vi "Edit Config.vi"(8 "error in (no error)":errorcluster, 11 "Lookup Table in":refnum<class "Lookup Table.lvclass">) -> (0 "error out":errorcluster, 3 "Lookup Table out":refnum<class "Lookup Table.lvclass">)   [LabVIEW 2018, in "Lookup Table.lvclass"]
doc: "Lookup Table.lvclass:Edit Config.vi\n\nThis VI is the configuration editor user interface for the Lookup Table class.\n\nInstrument Communication Module Version 1.0\nSeptember, 2017 Original Code Consulting David Thomson\n www.originalcode.com"
uses:
  Lookup Table.lvclass
  ICM Editor Command.ctl
  ICM Class Editor State.ctl
  ICM Config Command.ctl
  Lookup Table.lvclass/Lookup Table.ctl
panel:
  in  "Export":bool
  in  "Import":bool
  in  "New Instance":string
  in  "Delete":bool
  in  "Add":bool
  in  "Revert Scaling":bool
  in  "Table":cluster{"Raw Value":dbl, "Scaled Value":dbl}[](array[cluster])
  in  "Instance":u16(ring) items=["table", "hello"]
  in  "Save":bool
  # "To Add New Scaling Instance:\n1. Enter name in New Instance control to the right\n2. Click Add New Button\n3. Select Name in Instance control to the left\n4. Edit table below"
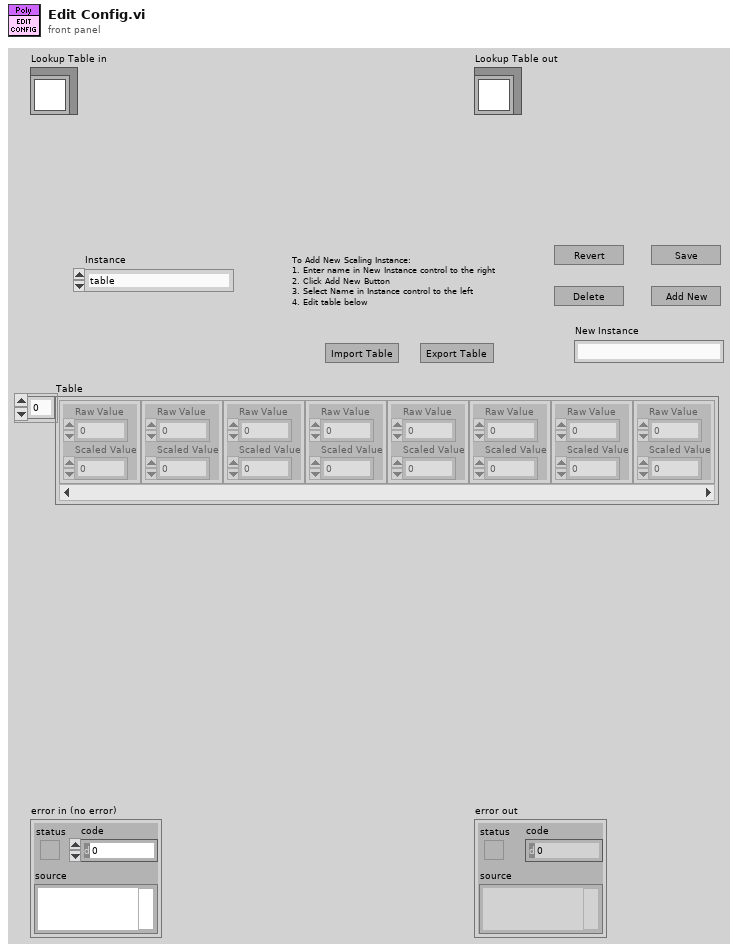
[diagram p1: front panel]
types:
  T1 = typedef "ICM Config Command.ctl" = enum16{"No-op", "Re-Display Sc."}
  T2 = typedef "ICM Class Editor State.ctl" = enum16{"Init", "Wait", "Write", "Read", "Display", "Set Flashing", "Error", "Stop"}
  T3 = typedef "ICM Editor Command.ctl" = enum16{"No-op", "Exit"}
  T4 = enum8{"Enabled", "Disabled", "Disabled and Grayed Out"}
  T5 = cluster{"Instance":string, "Table":cluster{"Raw Value":dbl, "Sca;ed Value":dbl}[]}
  T6 = cluster{"Instance":string, "Table":cluster{"Raw Value":dbl, "Scaled Value":dbl}[]}[]
  T7 = cluster{"RingText.Text":string, "Table":cluster{"Raw Value":dbl, "Scaled Value":dbl}[]}
  T8 = cluster{"Instance":string, "Table":cluster{"Raw Value":dbl, "Sca;ed Value":dbl}[]}[]
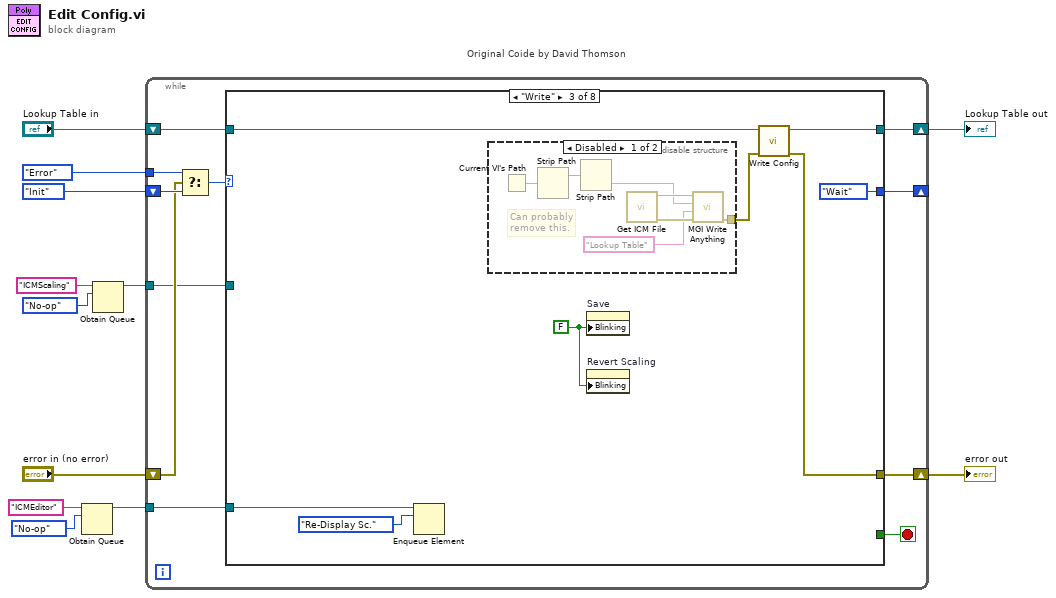
[diagram p0: block diagram]
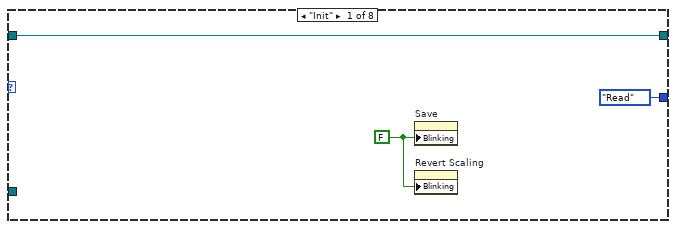
[diagram p2: hidden frame]
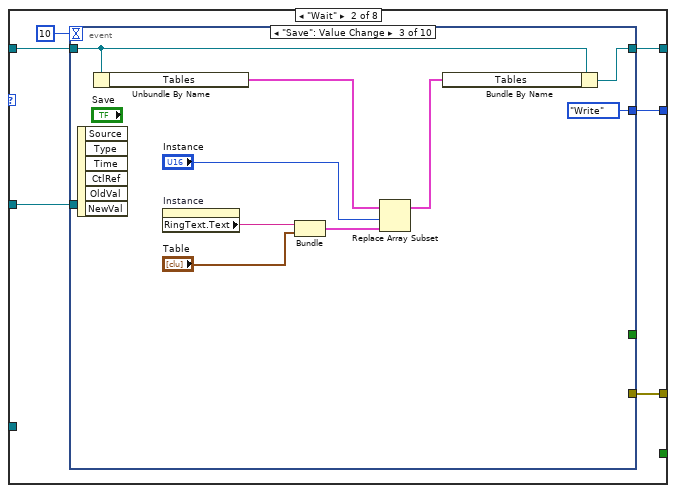
[diagram p3: hidden frame]
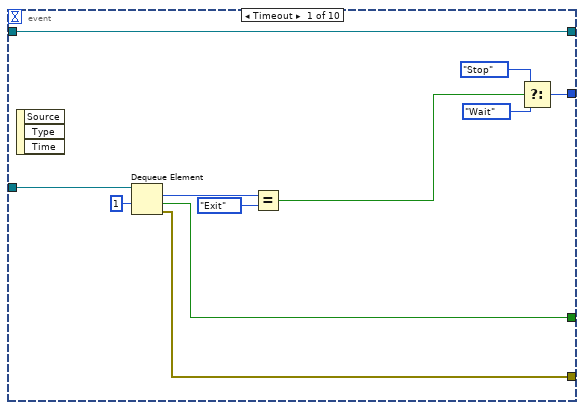
[diagram p4: hidden frame]
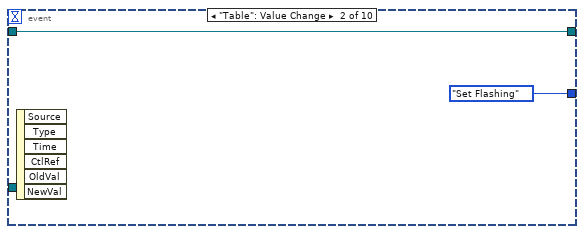
[diagram p5: hidden frame]
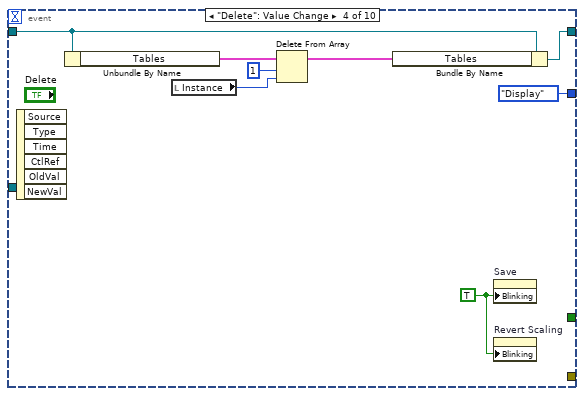
[diagram p6: hidden frame]
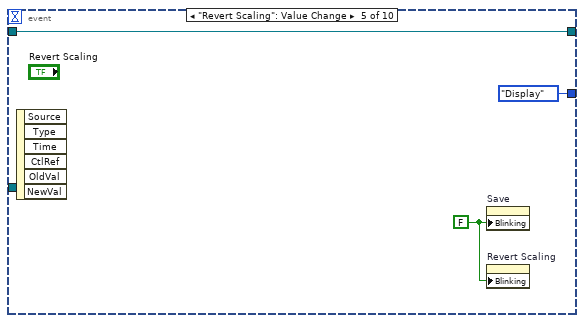
[diagram p7: hidden frame]
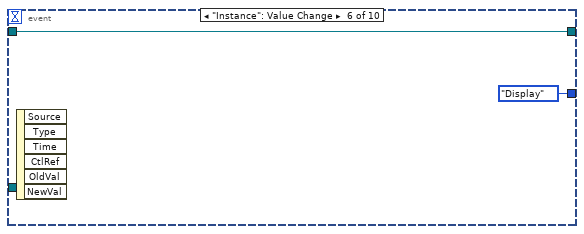
[diagram p8: hidden frame]
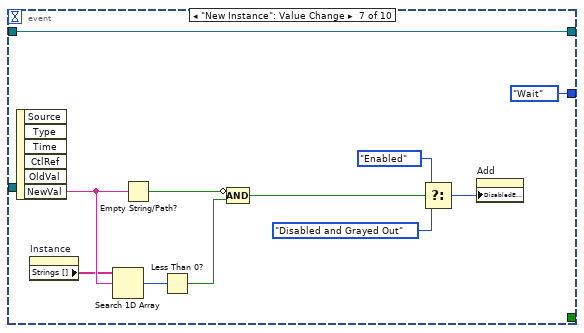
[diagram p9: hidden frame]
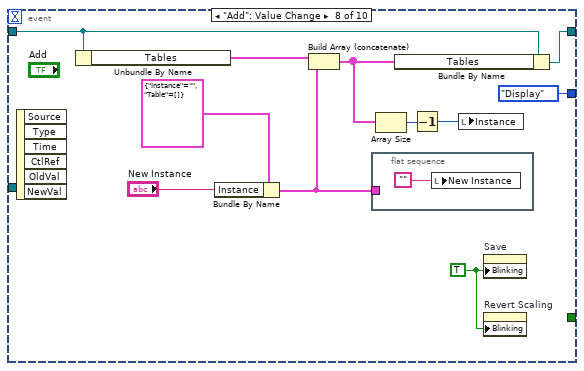
[diagram p10: hidden frame]
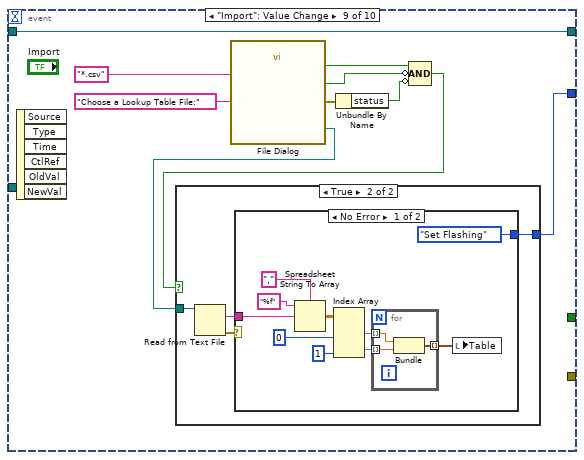
[diagram p11: hidden frame]
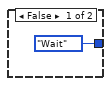
[diagram p12: hidden frame]
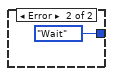
[diagram p13: hidden frame]
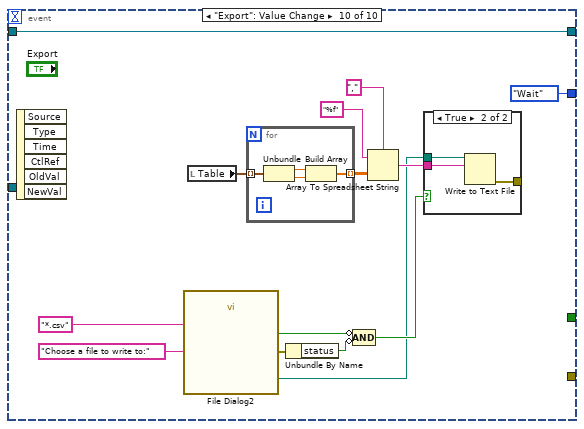
[diagram p14: hidden frame]
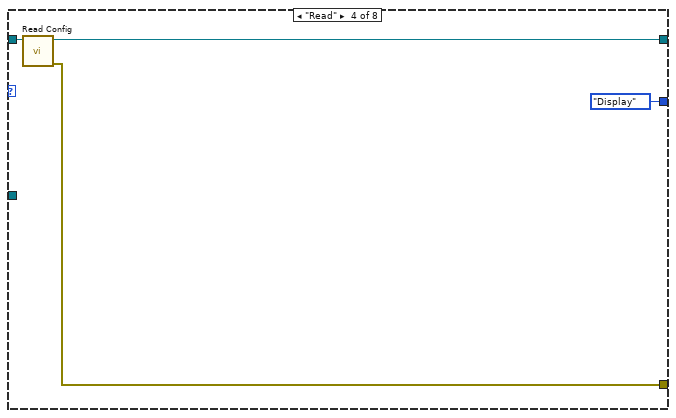
[diagram p17: hidden frame]
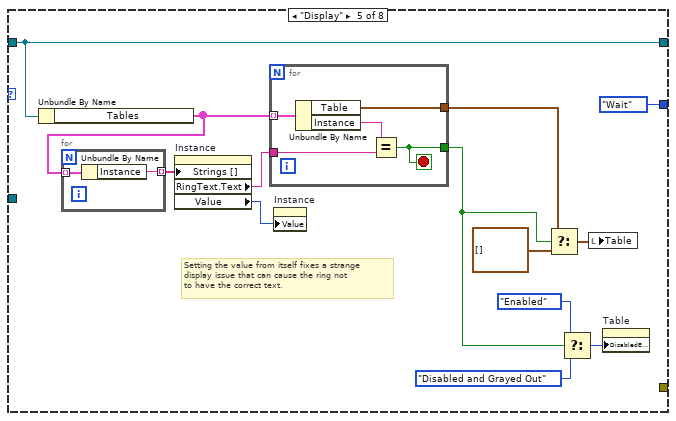
[diagram p18: hidden frame]
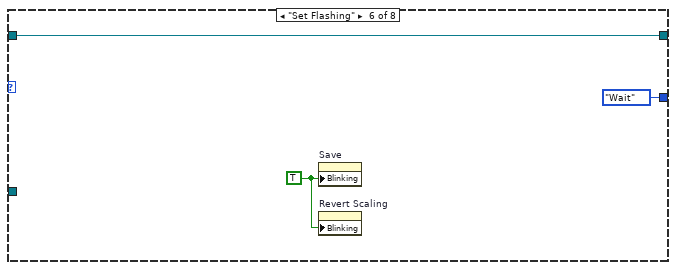
[diagram p19: hidden frame]
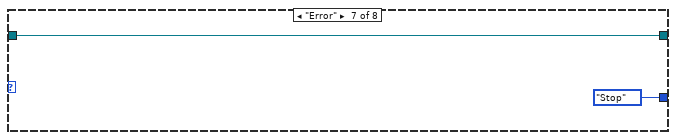
[diagram p20: hidden frame]
diagram:
  n1 = Obtain Queue(name (unnamed)="ICMEditor", element data type=ICM_Config_Command."No-op" ("Editor Command")) -> (queue out=w1:refnum<queue>)  [unwired: 3 in, 2 out]
  n2 = Obtain Queue(name (unnamed)="ICMScaling", element data type=ICM_Editor_Command."No-op" ("Editor Command")) -> (queue out=w8:refnum<queue>)  [unwired: 3 in, 2 out]
  n3 = while "Original Coide by David Thomson" {
    shift-right: [w23] -> w11
    shift-left: "Lookup Table in" -> [w22]
    shift-right: [w16] -> _
    shift-left: ICM_Class_Editor_State."Init" ("Config State") -> [w20]
    shift-right: [w15] -> w4
    shift-left: "error in (no error)" -> [w18]
    tunnel: ICM_Class_Editor_State."Error" ("Config State") -> [w17]
    tunnel: w8 -> [w14]
    tunnel: w1 -> [w13]
    stop <- w21 stop-if-true
    n4 = Select(t=w17, s=w18, f=w20) -> (s? t:f=w19:T2)
    n5 = case shown="\"Write\"" w19 {
      tunnel: [w25 w30 w147 w156 w168 w182 w184 w187] -> w23
      tunnel: w22 -> [w25 w29 w144 w158 w168 w182 w184 w187]
      tunnel: [_ _ _ _ _ _ _ TRUE] -> w21
      tunnel: [ICM_Class_Editor_State."Read" ("Config State") w31 ICM_Class_Editor_State."Wait" ("Config State") ICM_Class_Editor_State."Display" ("Config State") ICM_Class_Editor_State."Wait" ("Config State") ICM_Class_Editor_State."Wait" ("Config State") ICM_Class_Editor_State."Stop" ("Config State") ICM_Class_Editor_State."Stop" ("Config State")] -> w16
      tunnel: [_ w27 w146 w157 _ _ _ _] -> w15
      tunnel: w14 -> [_ w28 _ _ _ _ _ _]
      tunnel: w13 -> [_ _ w141 _ _ _ _ _]
      frame "Init" {
        w24 = FALSE ("Blinking")
        n6 = property on="Save" class="Bool"("Blinking"=w24) -> ()  [unwired: 2 in, 2 out]
        n7 = property on="Revert Scaling" class="Bool"("Blinking"=w24) -> ()  [unwired: 2 in, 2 out]
      }
      frame "Wait" {
        n8 = event shown="[2] \"Save\": Value Change" {
          selector: _ -> [_ _ _ _ _ _ _ _ _ _]
          dyn-events: _ -> [_ _ _ _ _ _ _ _ _ _]
          timeout: 10 -> [_ _ _ _ _ _ _ _ _ _]
          tunnel: [w40 ICM_Class_Editor_State."Set Flashing" ("Config State") ICM_Class_Editor_State."Write" ("Config State") ICM_Class_Editor_State."Display" ("Config State") ICM_Class_Editor_State."Display" ("Config State") ICM_Class_Editor_State."Display" ("Config State") ICM_Class_Editor_State."Wait" ("Config State") ICM_Class_Editor_State."Display" ("Config State") w91 ICM_Class_Editor_State."Wait" ("Config State")] -> w31
          tunnel: [w43 w45 w53 w57 w65 w67 w78 w87 w100 w133] -> w30
          tunnel: w29 -> [w43 w45 w52 w58 w65 w67 w78 w88 w100 w133]
          tunnel: w28 -> [w42 _ _ _ _ _ _ _ _ _]
          tunnel: [w34 _ _ _ _ _ _ _ _ _] -> w27
          tunnel: [w33 _ _ _ _ _ _ _ _ _] -> _
          event Timeout {
            n9 = event-data() -> ()  [unwired: 1 in, 3 out]
            n10 = Dequeue Element(queue=w42, timeout in ms (-1)=1) -> (element=w39:T3, timed out?=w33:bool, error out=w34:errorcluster)  [unwired: 1 in, 1 out]
            n11 = Equal?(x=w39, y=ICM_Editor_Command."Exit") -> (x = y?=w37:bool)
            n12 = Select(t=ICM_Class_Editor_State."Stop" ("Config State"), s=w37, f=ICM_Class_Editor_State."Wait" ("Config State")) -> (s? t:f=w40:T2)
          }
          event "Table": Value Change {
            n13 = event-data() -> ()  [unwired: 1 in, 6 out]
          }
          event "Save": Value Change {
            n14 = event-data() -> ()  [unwired: 1 in, 6 out]
            n15 = Unbundle By Name(w52) -> ("Tables"=w50:T6)
            n16 = property on="Instance" class="Ring (strict)"() -> ("RingText.Text"=w47:string)  [unwired: 2 in, 2 out]
            n17 = Bundle("RingText.Text"=w47, "Table"="Table") -> (w51:T7)  [unwired: 1 in]
            n18 = Replace Array Subset(array=w50, new element=w51, index="Instance") -> (w49:T6)
            n19 = Bundle By Name(cluster=w52, "Tables"=w49) -> (w53:refnum<class "Lookup Table.lvclass">)
          }
          event "Delete": Value Change {
            w62 = TRUE ("Blinking")
            n20 = event-data() -> ()  [unwired: 1 in, 6 out]
            n21 = Unbundle By Name(w58) -> ("Tables"=w59:T6)
            n22 = local read "Instance"() -> (w56:u16)
            n23 = Delete From Array(array=w59, length=1, index=w56) -> (array with subset deleted=w61:T6)  [unwired: 1 out]
            n24 = Bundle By Name(cluster=w58, "Tables"=w61) -> (w57:refnum<class "Lookup Table.lvclass">)
            n25 = property on="Save" class="Bool"("Blinking"=w62) -> ()  [unwired: 2 in, 2 out]
            n26 = property on="Revert Scaling" class="Bool"("Blinking"=w62) -> ()  [unwired: 2 in, 2 out]
          }
          event "Revert Scaling": Value Change {
            w63 = FALSE ("Blinking")
            n27 = event-data() -> ()  [unwired: 1 in, 6 out]
            n28 = property on="Save" class="Bool"("Blinking"=w63) -> ()  [unwired: 2 in, 2 out]
            n29 = property on="Revert Scaling" class="Bool"("Blinking"=w63) -> ()  [unwired: 2 in, 2 out]
          }
          event "Instance": Value Change {
            n30 = event-data() -> ()  [unwired: 1 in, 6 out]
          }
          event "New Instance": Value Change {
            n31 = event-data() -> ("NewVal"=w70:string)  [unwired: 1 in, 5 out]
            n32 = property on="Instance" class="Ring (strict)"() -> ("Strings []"=w68:string[])  [unwired: 2 in, 2 out]
            n33 = Search 1D Array(1D array=w68, element=w70) -> (index of element=w75:i32)  [unwired: 1 in]
            n34 = Empty String/Path?(string/path=w70) -> (empty?=w73:bool)
            n35 = Less Than 0?(x=w75) -> (x < 0?=w76:bool)
            n36 = Compound Arithmetic op=AND(invert w73, w76) -> (w74:bool)
            n37 = Select(t=T4."Enabled" ("Disabled"), s=w74, f=T4."Disabled and Grayed Out" ("Disabled")) -> (s? t:f=w69:T4)
            n38 = property on="Add" class="Bool"("DisabledEnum"=w69) -> ()  [unwired: 2 in, 2 out]
          }
          event "Add": Value Change {
            w83 = TRUE ("Blinking")
            n39 = event-data() -> ()  [unwired: 1 in, 6 out]
            n40 = Unbundle By Name(w88) -> ("Tables"=w89:T6)
            n41 = Bundle By Name(cluster=T5 {"Instance"="", "Table"=[]} ("Cluster"), "Instance"="New Instance") -> (w79:T5)
            n42 = Build Array (concatenate)(w89, w79) -> (w81:T8)
            n43 = flat-sequence {
              tunnel: w79 -> [_]
              frame #0 {
                n44 = local write "New Instance"("") -> ()
              }
            }
            n45 = Array Size(array=w81) -> (size(s)=w82:i32)
            n46 = Bundle By Name(cluster=w88, "Tables"=w81) -> (w87:refnum<class "Lookup Table.lvclass">)
            n47 = Decrement(x=w82) -> (x-1=w80:i32)
            n48 = local write "Instance"(w80) -> ()
            n49 = property on="Save" class="Bool"("Blinking"=w83) -> ()  [unwired: 2 in, 2 out]
            n50 = property on="Revert Scaling" class="Bool"("Blinking"=w83) -> ()  [unwired: 2 in, 2 out]
          }
          event "Import": Value Change {
            n51 = event-data() -> ()  [unwired: 1 in, 6 out]
            n52 = call "File Dialog"("prompt"="Choose a Lookup Table File:" ("prompt (Open existing file)"), "pattern (all files)"="*.csv") -> ("selected path"=w93:path, "exists"=w97:bool, "cancelled"=w96:bool, "error out"=w95:errorcluster)  [unwired: 10 in]
            n53 = Unbundle By Name(w95) -> ("status"=w94:bool)
            n54 = Compound Arithmetic op=AND(w97, invert w96, invert w94) -> (w92:bool)
            n55 = case shown="True" w92 {
              tunnel: w93 -> [_ w103]
              tunnel: [ICM_Class_Editor_State."Wait" ("Config State") w102] -> w91
              frame False {
              }
              frame True {
                n56 = Read from Text File(file (use dialog)=w103) -> (text=w105:string, error out=w104:errorcluster)  [unwired: 2 in, 3 out]
                n57 = case shown="No Error" w104 {
                  tunnel: w105 -> [w115 _]
                  tunnel: [ICM_Class_Editor_State."Set Flashing" ("Config State") ICM_Class_Editor_State."Wait" ("Config State")] -> w102
                  frame No Error {
                    n58 = Spreadsheet String To Array(delimiter (Tab)=",", format string="%f", spreadsheet string=w115) -> (array=w112:dbl[][])  [unwired: 1 out]
                    n59 = Index Array(array=w112, index (col) #1=0 ("disabled index (col)"), index (col) #2=1 ("index (col)")) -> (element #1=w109:dbl[], element #2=w108:dbl[])  [unwired: 2 in]
                    n60 = for {
                      tunnel: w109 -> [w117] mode=indexing
                      tunnel: w108 -> [w118] mode=indexing
                      tunnel: [w116] -> w106 mode=indexing
                      n61 = Bundle(w117, w118) -> (w116:cluster{dbl, dbl})  [unwired: 1 out]
                    }
                    n62 = local write "Table"(w106) -> ()
                  }
                  frame Error {
                  }
                }
              }
            }
          }
          event "Export": Value Change {
            n63 = event-data() -> ()  [unwired: 1 in, 6 out]
            n64 = call "File Dialog2"("prompt"="Choose a file to write to:" ("prompt (Open existing file)"), "pattern (all files)"="*.csv") -> ("selected path"=w120:path, "cancelled"=w124:bool, "error out"=w125:errorcluster)  [unwired: 10 in, 1 out]
            n65 = local read "Table"() -> (w128:cluster{"Raw Value":dbl, "Scaled Value":dbl}[])
            n66 = for {
              tunnel: w128 -> [w140] mode=indexing
              tunnel: [w137] -> w129 mode=indexing
              n67 = Unbundle(w140) -> ("Raw Value"=w139:dbl, "Scaled Value"=w138:dbl)
              n68 = Build Array(w139, w138) -> (w137:dbl[])
            }
            n69 = Unbundle By Name(w125) -> ("status"=w126:bool)
            n70 = Compound Arithmetic op=AND(invert w124, invert w126) -> (w121:bool)
            n71 = Array To Spreadsheet String(delimiter (Tab)=",", array=w129, 3:"%f" ("format string")) -> (spreadsheet string=w132:string)
            n72 = case shown="True" w121 {
              tunnel: w132 -> [_ w136]
              tunnel: w120 -> [_ w135]
              tunnel: [_ w134] -> _
              frame False {
              }
              frame True {
                n73 = Write to Text File(file (use dialog)=w135, text=w136) -> (error out=w134:errorcluster)  [unwired: 2 in, 2 out]
              }
            }
          }
        }
      }
      frame "Write" {
        w143 = FALSE ("Blinking")
        n74 = Enqueue Element(queue=w141, element=ICM_Config_Command."Re-Display Sc.") -> ()  [unwired: 2 in, 3 out]
        n75 = disable-structure shown="Disabled" {
          disable-tunnel: [w151 _] -> w145
          frame Disabled {
            # "Can probably\nremove this."
            n76 = Current VI's Path() -> (path=w155:path)
            n77 = Strip Path(path=w155) -> (stripped path=w154:path)  [unwired: 1 out]
            n78 = Strip Path(path=w154) -> (name=w150:string)  [unwired: 1 out]
            n79 = call "Get ICM File.vi"() -> ("error out"=w152:errorcluster, "ICM File"=w153:path)  [unwired: 10 in]
            n80 = call "MGI Write Anything.vi"("Error In"=w152, "Section Name (Name of \"Anything\")"="Lookup Table" ("Section Name (Name of \"Anything\")"), "Anything"=w150, "Path (dialog)"=w153) -> ("Error Out"=w151:errorcluster)  [unwired: 5 in, 2 out]
          }
          frame Enabled {
          }
        }
        n81 = property on="Save" class="Bool"("Blinking"=w143) -> ()  [unwired: 2 in, 2 out]
        n82 = property on="Revert Scaling" class="Bool"("Blinking"=w143) -> ()  [unwired: 2 in, 2 out]
        n83 = call-dynamic "Write Config.vi"("error in (no error)"=w145, "Lookup Table in"=w144) -> ("error out"=w146:errorcluster, "Lookup Table out"=w147:refnum<class "Lookup Table.lvclass">)  [unwired: 8 in]
      }
      frame "Read" {
        n84 = call-dynamic "Read Config.vi"("Lookup Table in"=w158) -> ("error out"=w157:errorcluster, "Lookup Table out"=w156:refnum<class "Lookup Table.lvclass">)  [unwired: 9 in]
      }
      frame "Display" {
        # "Setting the value from itself fixes a strange\ndisplay issue that can cause the ring not\nto have the correct text."
        n85 = Unbundle By Name(w168) -> ("Tables"=w167:T6)
        n86 = for {
          tunnel: w167 -> [w174] mode=indexing
          tunnel: [w173] -> w166 mode=indexing
          n87 = Unbundle By Name(w174) -> ("Instance"=w173:string)
        }
        n88 = property on="Instance" class="Ring (strict)"("Strings []"=w166) -> ("RingText.Text"=w165:string, "Value"=w160:u16)  [unwired: 2 in, 2 out]
        n89 = for {
          tunnel: w167 -> [w179] mode=indexing
          tunnel: w165 -> [w177]
          tunnel: [w176] -> w161
          tunnel: [w175] -> w171
          stop <- w176 stop-if-true
          n90 = Unbundle By Name(w179) -> ("Table"=w175:cluster{"Raw Value":dbl, "Scaled Value":dbl}[], "Instance"=w178:string)
          n91 = Equal?(x=w178, y=w177) -> (x = y?=w176:bool)
        }
        n92 = property on="Instance" class="Ring (strict)"("Value"=w160) -> ()  [unwired: 2 in, 2 out]
        n93 = Select(t=w171, s=w161, f=cluster{"Raw Value":dbl, "Sca;ed Value":dbl}[] []) -> (s? t:f=w169:cluster{"Raw Value":dbl, "Sca;ed Value":dbl}[])
        n94 = Select(t=T4."Enabled" ("Disabled"), s=w161, f=T4."Disabled and Grayed Out" ("Disabled")) -> (s? t:f=w162:T4)
        n95 = local write "Table"(w169) -> ()
        n96 = property on="Table" class="Arr (strict)"("DisabledEnum"=w162) -> ()  [unwired: 2 in, 2 out]
      }
      frame "Set Flashing" {
        w180 = TRUE ("Blinking")
        n97 = property on="Save" class="Bool"("Blinking"=w180) -> ()  [unwired: 2 in, 2 out]
        n98 = property on="Revert Scaling" class="Bool"("Blinking"=w180) -> ()  [unwired: 2 in, 2 out]
      }
      frame "Error" {
      }
      frame "Stop" {
      }
    }
  }
  "error out" <- w4
  "Lookup Table out" <- w11
